vi "Adv_GetROI.vi"(6 "error in (no error)":errorcluster, 11 "LightField Automation in":refnum<class "LightField Automation.lvclass">) -> (0 "YBinning":i32, 1 "XBinning":i32, 2 "Width":i32, 3 "LightField Automation out":refnum<class "LightField Automation.lvclass">, 4 "error out":errorcluster, 8 "Y":i32, 9 "X":i32, 10 "Height":i32)   [LabVIEW 2019, in "LightField Automation.lvclass"]
uses:
  LightField Automation.lvclass
  LightField Automation.lvclass/LightField Automation.ctl
  C:/Program Files/Princeton Instruments/LightField/AddInViews/PrincetonInstruments.LightFieldViewV3.dll
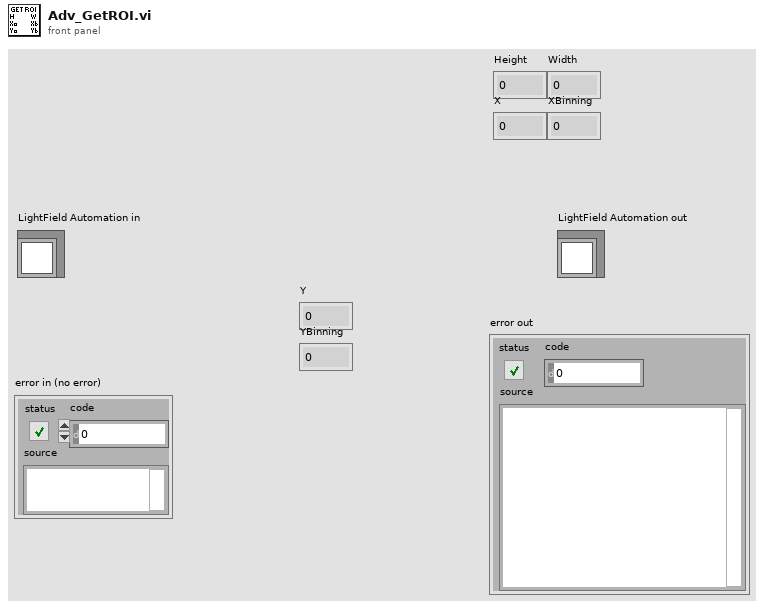
[diagram p1: front panel]
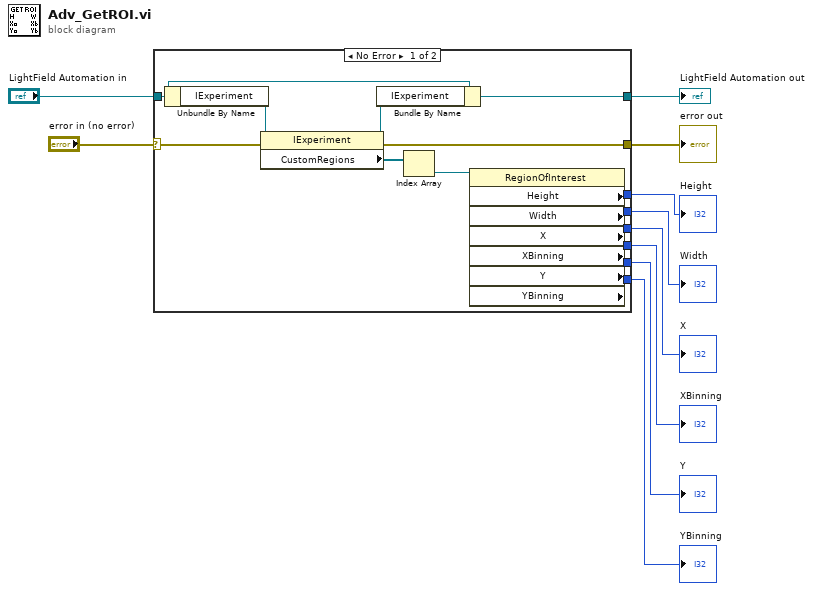
[diagram p0: block diagram]
diagram:
  n1 = case shown="No Error" "error in (no error)" {
    selector: "error in (no error)" -> [w23 w26]
    tunnel: "LightField Automation in" -> [w17 w25]
    tunnel: [w16 w25] -> w9
    tunnel: [w18 w26] -> w7
    tunnel: [w20 _] -> w6
    tunnel: [w19 _] -> w5
    tunnel: [w14 _] -> w4
    tunnel: [w13 _] -> w3
    tunnel: [w12 _] -> w2
    tunnel: [w11 _] -> w1
    frame No Error {
      n2 = Unbundle By Name(w17) -> ("IExperiment"=w24:refnum<k24>)
      n3 = property class="IExperiment"(reference=w24, error in=w23) -> (reference out=w15:refnum<k24>, error out=w18:errorcluster, "CustomRegions"=w22:refnum<k24>[])
      n4 = Bundle By Name(cluster=w17, "IExperiment"=w15) -> (w16:refnum<class "LightField Automation.lvclass">)
      n5 = Index Array(array=w22) -> (element=w21:refnum<k24>)  [unwired: 1 in]
      n6 = property class="RegionOfInterest"(reference=w21) -> ("Height"=w20:i32, "Width"=w19:i32, "X"=w14:i32, "XBinning"=w13:i32, "Y"=w12:i32, "YBinning"=w11:i32)  [unwired: 1 in, 2 out]
    }
    frame Error {
    }
  }
  "LightField Automation out" <- w9
  "error out" <- w7
  "Y" <- w2
  "YBinning" <- w1
  "Height" <- w6
  "Width" <- w5
  "X" <- w4
  "XBinning" <- w3
